vi "DWF FGEN Query Arbitrary Waveform Gain and Offset.vi"(0 "Instrument Handle In":u32, 11 "Error In":errorcluster caption="Error In (no error)") -> (4 "Instrument Handle Out":u32, 6 "Gain":dbl, 8 "Offset":dbl, 15 "Error Out":errorcluster)   [LabVIEW 2015, in "DigilentWF.lvlib"]
doc: "Returns the settings for arbitrary waveform generation that includes gain and offset settings."
uses:
  <vilib>/DigilentWF/DigilentWF.lvlib
  dwf.dll
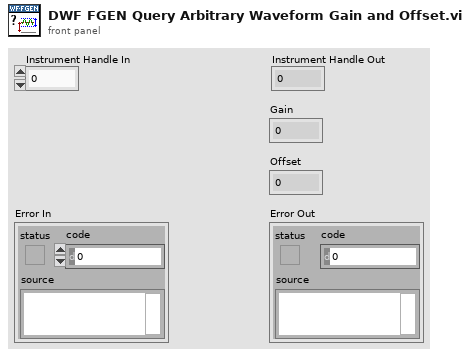
[diagram p1: front panel]
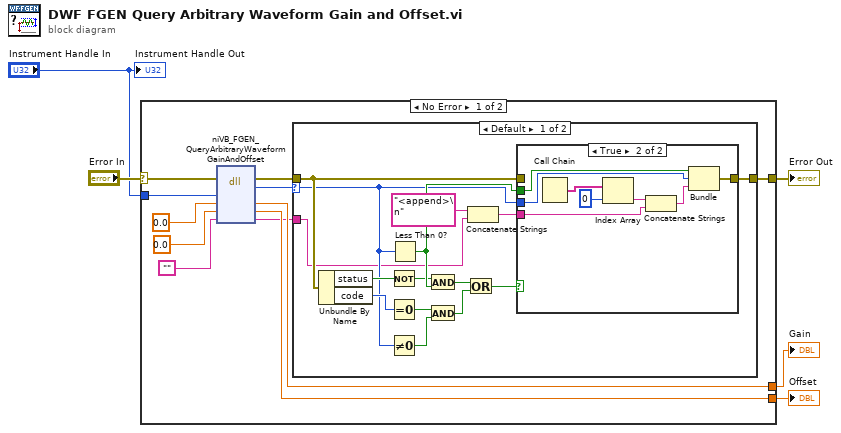
[diagram p0: block diagram]
diagram:
  n1 = case "outter_case" shown="No Error" "Error In" {
    selector: "Error In" -> [w16 w42]
    tunnel: [w13 w42] -> w4
    tunnel: "Instrument Handle In" -> [w12 _]
    tunnel: [w9 _] -> w2
    tunnel: [w8 _] -> w1
    frame No Error {
      n2 = dll-call lib="dwf.*" fn="niVB_FGEN_QueryArbitraryWaveformGainAndOffset"(error in=w16, "InstrumentHandle"=w12, "Gain"=0.0, "Offset"=0.0, "szError"="") -> (error out=w15:errorcluster, "return type"=w14:i32, "Gain"=w9:dbl, "Offset"=w8:dbl, "szError"=w6:string)  [unwired: 3 in, 1 out]
      n3 = case "inner_case" shown="Default" w14 {
        selector: w14 -> [w21 _]
        tunnel: w15 -> [w22 w41]
        tunnel: [w18 w41] -> w13
        tunnel: w6 -> [w17 _]
        frame Default {
          n4 = Unbundle By Name(w22) -> ("status"=w26:bool, "code"=w30:i32)
          n5 = Not(x=w26) -> (.not. x?=w29:bool)
          n6 = Equal To 0?(x=w30) -> (x = 0?=w25:bool)
          n7 = Not Equal To 0?(x=w21) -> (x != 0?=w28:bool)
          n8 = Less Than 0?(x=w21) -> (x < 0?=w31:bool)
          n9 = And(x=w29, y=w31) -> (x .and. y?=w27:bool)
          n10 = And(x=w25, y=w28) -> (x .and. y?=w24:bool)
          n11 = Or(x=w27, y=w24) -> (x .or. y?=w23:bool)
          n12 = Concatenate Strings("<append>\n" ("string"), w17) -> (w20:string)
          n13 = case shown="True" w23 {
            tunnel: [w32 w39] -> w18
            tunnel: w21 -> [_ w38]
            tunnel: w31 -> [_ w37]
            tunnel: w22 -> [w32 _]
            tunnel: w20 -> [_ w33]
            frame False {
            }
            frame True {
              n14 = Call Chain() -> (call chain=w36:string[])
              n15 = Index Array(array=w36, index=0) -> (element=w35:string)
              n16 = Concatenate Strings(w35, w33) -> (w40:string)
              n17 = Bundle(w37, "return type"=w38, w40) -> (w39:cluster{bool, "return type":i32, string})  [unwired: 1 out]
            }
          }
        }
        frame 0 {
        }
      }
    }
    frame Error {
    }
  }
  "Error Out" <- w4
  "Gain" <- w2
  "Offset" <- w1
  "Instrument Handle Out" <- "Instrument Handle In"
